vi "Read Line Rate - With One Method - Returns Total Value.vi"() -> ()   [LabVIEW 2017, in "Cobertura.Tests.lvlib" / "Coverage.lvlib"]
uses:
  Coverage.lvlib
  Cobertura/Coverage/Coverage.lvclass/Coverage.ctl
  Cobertura/Coverage/Read Line Rate.vi
  <vilib>/PNR/Transparent Assertions/Transparent Assertions/Transparent Assertions.lvlib
  Cobertura/Package/Package.lvclass
  Cobertura/Class/Class.lvclass
  Cobertura/Method/Method.lvclass
  Cobertura/Coverage/Coverage.lvclass
panel:
  out "error out":errorcluster
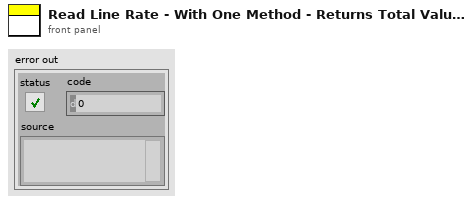
[diagram p1: front panel]
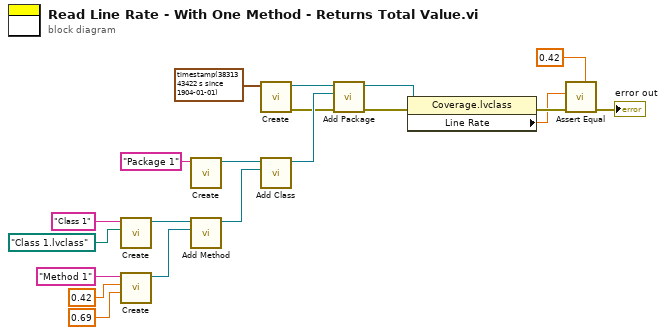
[diagram p0: block diagram]
diagram:
  n1 = call "Create.vi"("Filename"=path "Class 1.lvclass", "Name"="Class 1") -> ("Class"=w17:refnum<class "Class.lvclass">)  [unwired: 8 in, 1 out]
  n2 = call "Create.vi"("Branch Rate"=0.69, "Line Rate"=0.42, "Name"="Method 1") -> ("Method"=w13:refnum<class "Method.lvclass">)  [unwired: 7 in, 1 out]
  n3 = call "Create.vi"("Name"="Package 1") -> ("Package"=w9:refnum<class "Package.lvclass">)  [unwired: 9 in, 1 out]
  n4 = call "Add Method.vi"("Method"=w13, "Class in"=w17) -> ("Class out"=w2:refnum<class "Class.lvclass">)  [unwired: 8 in, 1 out]
  n5 = call "Create.vi"("Timestamp"=timestamp(3831343422.3303647 s since 1904-01-01)) -> ("error out"=w5:errorcluster, "Coverage"=w8:refnum<class "Coverage.lvclass">)  [unwired: 9 in]
  n6 = call "Add Class.vi"("Class"=w2, "Package in"=w9) -> ("Package out"=w6:refnum<class "Package.lvclass">)  [unwired: 8 in, 1 out]
  n7 = call "Add Package.vi"("error in (no error)"=w5, "Package"=w6, "Coverage in"=w8) -> ("error out"=w7:errorcluster, "Coverage out"=w4:refnum<class "Coverage.lvclass">)  [unwired: 7 in]
  n8 = property class="Coverage.lvclass"(reference=w4, error in=w7) -> (error out=w19:errorcluster, "Line Rate"=w12:dbl)  [unwired: 1 out]
  n9 = call <vilib>:"Assert Equal.vi"("Expected"=0.42 ("Branch Rate"), "error in (no error)"=w19, "Actual"=w12) -> ("error out"=→"error out":errorcluster)  [unwired: 8 in]
